vi "Test Queue Operations.vi"() -> ()   [LabVIEW 2013]
uses:
  ByteFIFO/ByteFIFO.lvclass
  VariantBuffer/VariantBuffer.lvclass
panel:
  out "read element ordering 2":bool
  out "read element ordering":bool
  out "disallowed overflow":bool
  out "15 element overflow":u8[](array[numeric]) format="%02x"
  out "previewed elements at index":bool
  out "index2 byte":u8 format="%02x"
  out "flushed":u8[](array[numeric]) format="%02x"
  out "5 element overflow":u8[](array[numeric]) format="%02x"
  out "10 more element overflow":u8[](array[numeric]) format="%02x"
  out "queue ten elements (array)":bool
  out "overflow enqueue >> bufSize":bool
  out "dequeued elements 2":bool
  out "last 5 elements":u8[](array[numeric]) format="%02x"
  out "dequeued":u8[](array[numeric]) format="%02x"
  out "dequeued elements":bool
  out "all elements read before destruction":bool
  out "queue ten elements (array)":bool
  out "returned all elements on destruction":bool
  out "overflow":u8[](array[numeric]) format="%02x"
  out "overflowed element retrieved":bool
  out "overflow loss an element":bool
  out "bufSize element - overflow":bool
  out "bufSize -1 element - no overflow":bool
  out "post-flush nbElements":bool
  out "error out":errorcluster
  out "flush return element count":bool
  out "last element matches":bool
  out "queue three elements -no overflow":bool
  out "queue three elements":bool
  out "last element found":bool
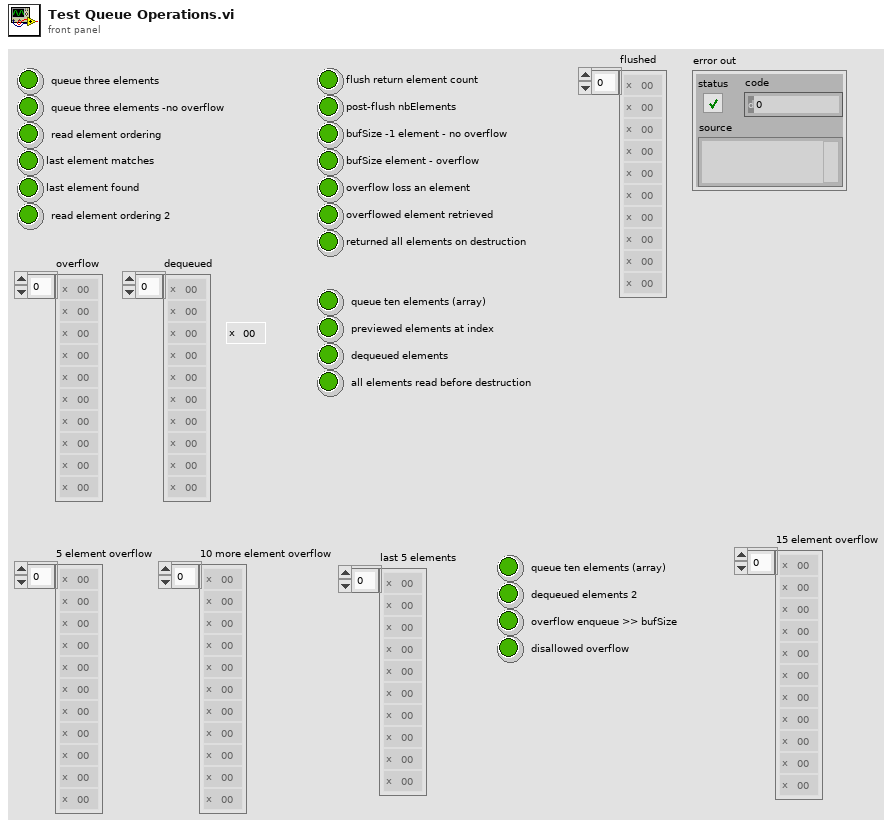
[diagram p1: front panel]
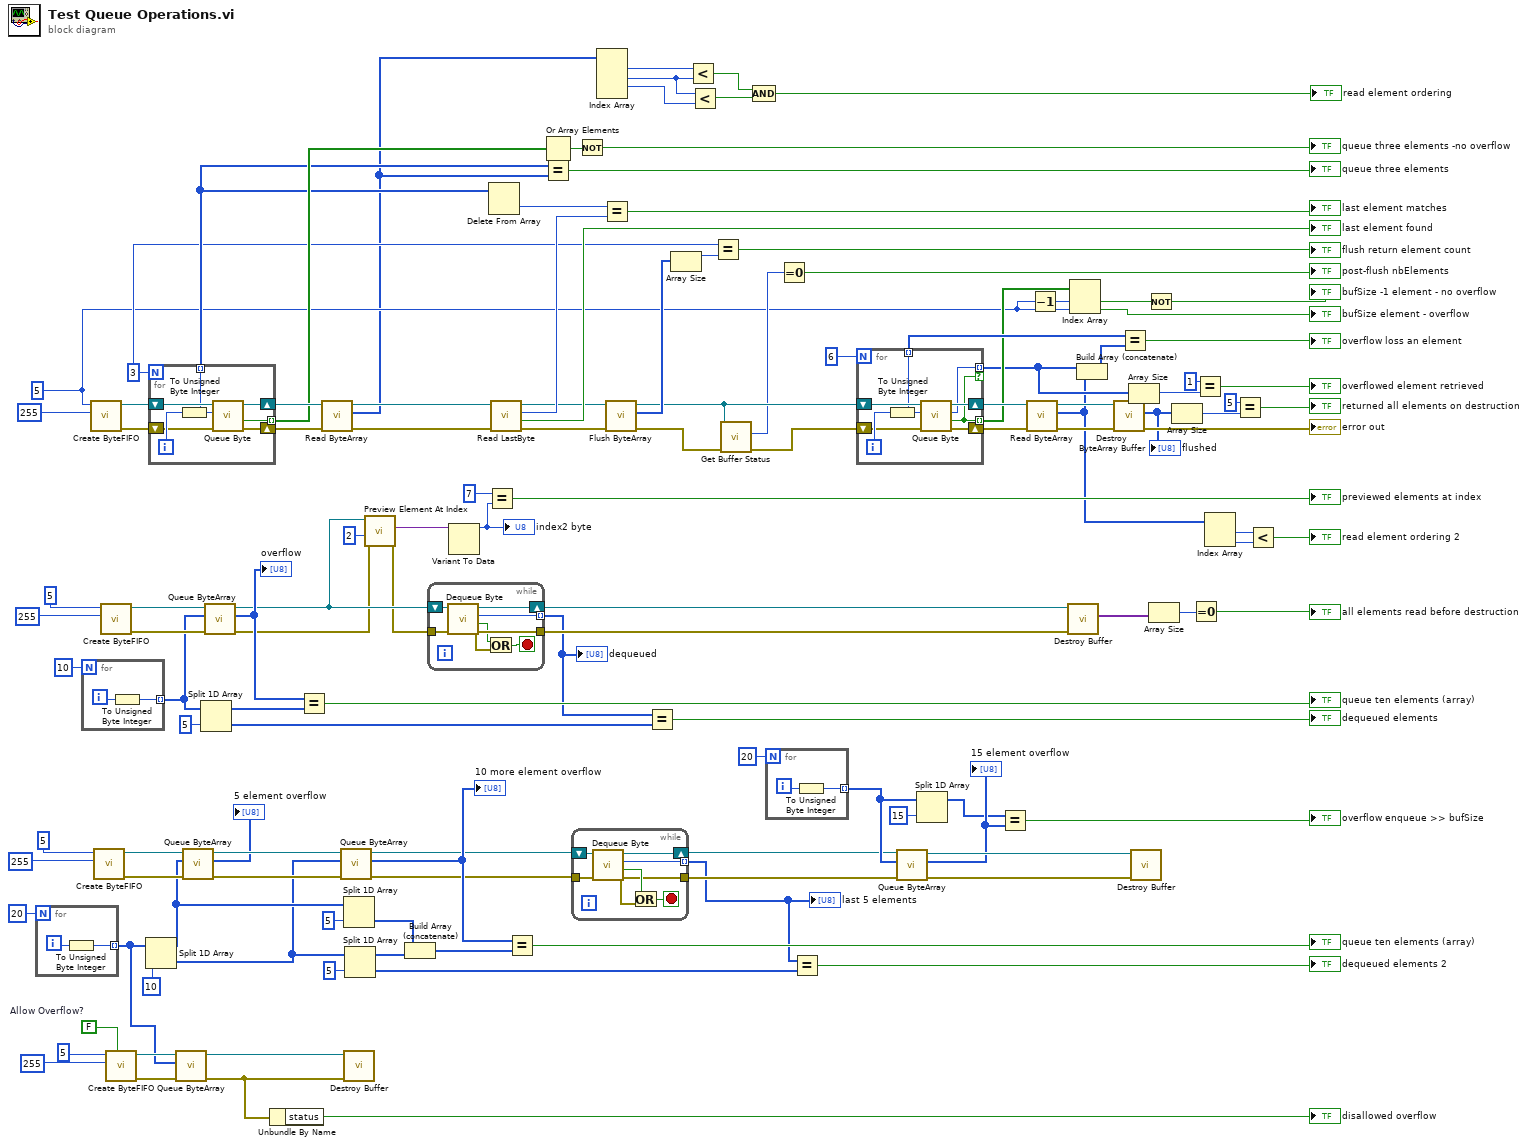
[diagram p0: block diagram]
diagram:
  w19 = FALSE  # Allow Overflow?
  w112 = 3
  w95 = 5 ("bufSize")
  n1 = for {
    N: 20 -> [_]
    tunnel: [w130] -> w16 mode=indexing
    i -> [w131]
    n2 = To Unsigned Byte Integer(number=w131) -> (unsigned 8bit integer=w130:u8)
  }
  n3 = for {
    N: 10 -> [_]
    tunnel: [w132] -> w72 mode=indexing
    i -> [w133]
    n4 = To Unsigned Byte Integer(number=w133) -> (unsigned 8bit integer=w132:u8)
  }
  n5 = call "Create ByteFIFO.vi"("default value"=u8 255, "bufSize"=w95) -> ("error out"=w109:errorcluster, "Buffer"=w128:refnum<data-value>)  [unwired: 8 in]
  n6 = call "Create ByteFIFO.vi"("default value"=u8 255, "bufSize"=5) -> ("error out"=w55:errorcluster, "Buffer"=w53:refnum<data-value>)  [unwired: 8 in]
  n7 = call "Create ByteFIFO.vi"("default value"=u8 255, "bufSize"=5) -> ("error out"=w80:errorcluster, "Buffer"=w81:refnum<data-value>)  [unwired: 8 in]
  n8 = call "Create ByteFIFO.vi"("Allow Overflow? (T)"=w19, "default value"=u8 255, "bufSize"=5) -> ("error out"=w17:errorcluster, "Buffer"=w18:refnum<data-value>)  [unwired: 7 in]
  n9 = Split 1D Array(array=w16, index=10) -> (first subarray=w45:u8[], second subarray=w43:u8[])
  n10 = for {
    N: w112 -> [_]
    shift-right: [w138] -> w127
    shift-left: w128 -> [w140]
    tunnel: [w137] -> w119 mode=indexing
    tunnel: [w136] -> w123 mode=indexing
    shift-right: [w134] -> w108
    shift-left: w109 -> [w135]
    i -> [w139]
    n11 = To Unsigned Byte Integer(number=w139) -> (unsigned 8bit integer=w137:u8)
    n12 = call "Queue Byte.vi"("error in"=w135, "byte"=w137, "Buffer"=w140) -> ("error out"=w134:errorcluster, "overflowed?"=w136:bool, "Buffer"=w138:refnum<data-value>)  [unwired: 5 in, 1 out]
  }
  n13 = call "Queue ByteArray.vi"("error in"=w17, "bytes"=w16, "Buffer"=w18) -> ("error out"=w14:errorcluster, "Buffer"=w15:refnum<data-value>)  [unwired: 6 in, 1 out]
  n14 = call "Queue ByteArray.vi"("error in"=w55, "bytes"=w45, "Buffer"=w53) -> ("error out"=w54:errorcluster, "overflow"=→"5 element overflow":u8[], "Buffer"=w52:refnum<data-value>)  [unwired: 6 in]
  n15 = Split 1D Array(array=w72, index=5) -> (first subarray=w66:u8[], second subarray=w65:u8[])
  n16 = call "Queue ByteArray.vi"("error in"=w80, "bytes"=w72, "Buffer"=w81) -> ("error out"=w40:errorcluster, "overflow"=w73:u8[], "Buffer"=w41:refnum<data-value>)  [unwired: 6 in]
  "overflow" <- w73
  n17 = Unbundle By Name(w14) -> ("status"=→"disallowed overflow":bool)
  n18 = Equal?(x=w73, y=w66) -> (x = y?=→"queue ten elements (array)":bool)
  n19 = call "Read ByteArray.vi"("error in"=w108, "Buffer"=w127) -> ("error out"=w107:errorcluster, "bytes"=w2:u8[], "Buffer"=w126:refnum<data-value>)  [unwired: 7 in]
  n20 = call "Queue ByteArray.vi"("error in"=w54, "bytes"=w43, "Buffer"=w52) -> ("error out"=w58:errorcluster, "overflow"=w59:u8[], "Buffer"=w21:refnum<data-value>)  [unwired: 6 in]
  "10 more element overflow" <- w59
  n21 = Split 1D Array(array=w45, index=5) -> (second subarray=w44:u8[])  [unwired: 1 out]
  n22 = call "Destroy Buffer.vi"("error in"=w14, "Buffer"=w15) -> ()  [unwired: 8 in, 2 out]
  n23 = Split 1D Array(array=w43, index=5) -> (first subarray=w48:u8[], second subarray=w62:u8[])
  n24 = call "Preview Element At Index.vi"("error in"=w40, "index (-1: last)"=2, "Buffer in"=w41) -> ("error out"=w39:errorcluster, "element"=w37:variant)  [unwired: 5 in, 2 out]
  n25 = Build Array (concatenate)(w44, w48) -> (w47:u8[])
  n26 = while {
    tunnel: w39 -> [w145]
    tunnel: [w143] -> w77
    tunnel: [w144] -> w12 mode=indexing
    shift-right: [w146] -> w78
    shift-left: w41 -> [w147]
    stop <- w141 stop-if-true
    n27 = call "Dequeue Byte.vi"("error in"=w145, "Buffer"=w147) -> ("error out"=w143:errorcluster, "buffer empty?"=w142:bool, "byte"=w144:u8, "Buffer"=w146:refnum<data-value>)  [unwired: 6 in]
    n28 = Or(x=w142, y=w143) -> (x .or. y?=w141:bool)
  }
  "dequeued" <- w12
  n29 = Variant To Data(Variant=w37) -> (data=w36:u8)  [unwired: 2 in, 1 out]
  "index2 byte" <- w36
  n30 = Equal?(x=u8 7, y=w36) -> (x = y?=→"previewed elements at index":bool)
  n31 = Delete From Array(array=w119) -> (deleted portion=w118:u8)  [unwired: 2 in, 1 out]
  n32 = call "Read LastByte.vi"("error in"=w107, "Buffer"=w126) -> ("error out"=w106:errorcluster, "found"=→"last element found":bool, "byte"=w120:u8, "Buffer"=w115:refnum<data-value>)  [unwired: 6 in]
  n33 = Equal?(x=w59, y=w47) -> (x = y?=→"queue ten elements (array)":bool)
  n34 = Or Array Elements(Boolean array=w123) -> (logical OR=w122:bool)
  n35 = Equal?(x=w119, y=w2) -> (x = y?=→"queue three elements":bool)
  n36 = while {
    tunnel: w58 -> [w153]
    tunnel: [w148] -> w31
    tunnel: [w152] -> w22 mode=indexing
    shift-right: [w151] -> w20
    shift-left: w21 -> [w154]
    stop <- w150 stop-if-true
    n37 = call "Dequeue Byte.vi"("error in"=w153, "Buffer"=w154) -> ("error out"=w148:errorcluster, "buffer empty?"=w149:bool, "byte"=w152:u8, "Buffer"=w151:refnum<data-value>)  [unwired: 6 in]
    n38 = Or(x=w149, y=w148) -> (x .or. y?=w150:bool)
  }
  "last 5 elements" <- w22
  n39 = Not(x=w122) -> (.not. x?=→"queue three elements -no overflow":bool)
  n40 = Index Array(array=w2) -> (element #1=w7:u8, element #2=w6:u8, element #3=w5:u8)  [unwired: 4 in, 1 out]
  n41 = Equal?(x=w118, y=w120) -> (x = y?=→"last element matches":bool)
  n42 = call "Flush ByteArray.vi"("error in"=w106, "Buffer"=w115) -> ("error out"=w105:errorcluster, "bytes"=w114:u8[], "Buffer"=w110:refnum<data-value>)  [unwired: 7 in]
  n43 = Equal?(x=w12, y=w65) -> (x = y?=→"dequeued elements":bool)
  n44 = Array Size(array=w114) -> (size(s)=w113:i32)
  n45 = Less?(x=w7, y=w6) -> (x < y?=w3:bool)
  n46 = Less?(x=w6, y=w5) -> (x < y?=w4:bool)
  n47 = Equal?(x=w112, y=w113) -> (x = y?=→"flush return element count":bool)
  n48 = call "Get Buffer Status.vi"("error in"=w105, "Buffer in"=w110) -> ("error out"=w104:errorcluster, "nbElements"=w102:i32)  [unwired: 5 in, 3 out]
  n49 = Compound Arithmetic op=AND(w3, w4) -> (→"read element ordering":bool)
  n50 = for {
    N: 20 -> [_]
    tunnel: [w155] -> w28 mode=indexing
    i -> [w156]
    n51 = To Unsigned Byte Integer(number=w156) -> (unsigned 8bit integer=w155:u8)
  }
  n52 = Equal To 0?(x=w102) -> (x = 0?=→"post-flush nbElements":bool)
  n53 = Equal?(x=w22, y=w62) -> (x = y?=→"dequeued elements 2":bool)
  n54 = for {
    N: 6 -> [_]
    shift-right: [w162] -> w98
    shift-left: w110 -> [w164]
    tunnel: [w159] -> w100 mode=indexing
    tunnel: [w157] -> w97 mode=indexing
    shift-right: [w160] -> w99
    shift-left: w104 -> [w161]
    tunnel: [w158] -> w89 mode=indexing if=w157
    i -> [w163]
    n55 = To Unsigned Byte Integer(number=w163) -> (unsigned 8bit integer=w159:u8)
    n56 = call "Queue Byte.vi"("error in"=w161, "byte"=w159, "Buffer"=w164) -> ("error out"=w160:errorcluster, "overflowed?"=w157:bool, "overflow"=w158:u8, "Buffer"=w162:refnum<data-value>)  [unwired: 5 in]
  }
  n57 = call "Queue ByteArray.vi"("error in"=w31, "bytes"=w28, "Buffer"=w20) -> ("error out"=w32:errorcluster, "overflow"=w27:u8[], "Buffer"=w33:refnum<data-value>)  [unwired: 6 in]
  "15 element overflow" <- w27
  n58 = Split 1D Array(array=w28, index=15) -> (first subarray=w25:u8[])  [unwired: 1 out]
  n59 = Equal?(x=w25, y=w27) -> (x = y?=→"overflow enqueue >> bufSize":bool)
  n60 = call "Read ByteArray.vi"("error in"=w99, "Buffer"=w98) -> ("error out"=w84:errorcluster, "bytes"=w9:u8[], "Buffer"=w85:refnum<data-value>)  [unwired: 7 in]
  n61 = Decrement(x=w95) -> (x-1=w96:i32)
  n62 = call "Destroy Buffer.vi"("error in"=w77, "Buffer"=w78) -> ("elements"=w69:variant[])  [unwired: 8 in, 1 out]
  n63 = Index Array(array=w97, index #1=w96, index #2=w95) -> (element #1=w94:bool, element #2=→"bufSize element - overflow":bool)
  n64 = Build Array (concatenate)(w89, w9) -> (w91:u8[])
  n65 = call "Destroy ByteArray Buffer.vi"("error in"=w84, "Buffer"=w85) -> ("error out"=→"error out":errorcluster, "bytes"=w42:u8[])  [unwired: 8 in]
  "flushed" <- w42
  n66 = Equal?(x=w100, y=w91) -> (x = y?=→"overflow loss an element":bool)
  n67 = Array Size(array=w89) -> (size(s)=w90:i32)
  n68 = call "Destroy Buffer.vi"("error in"=w32, "Buffer"=w33) -> ()  [unwired: 8 in, 2 out]
  n69 = Not(x=w94) -> (.not. x?=→"bufSize -1 element - no overflow":bool)
  n70 = Array Size(array=w69) -> (size(s)=w68:i32)
  n71 = Array Size(array=w42) -> (size(s)=w75:i32)
  n72 = Equal To 0?(x=w68) -> (x = 0?=→"all elements read before destruction":bool)
  n73 = Equal?(x=1, y=w90) -> (x = y?=→"overflowed element retrieved":bool)
  n74 = Index Array(array=w9) -> (element #1=w10:u8, element #2=w11:u8)  [unwired: 2 in]
  n75 = Equal?(x=5, y=w75) -> (x = y?=→"returned all elements on destruction":bool)
  n76 = Less?(x=w10, y=w11) -> (x < y?=→"read element ordering 2":bool)
